vi "Config Select.vi"(0 "Config Dir":path=path "C:/Users/gtetil/Documents/Projects/TI-cDAQ/Source/Support/Configurations", 1 "Config Extension":string="*.std", 5 "Error IN":errorcluster) -> (14 "Load Config":bool, 15 "Config Name":string, 19 "Error OUT":errorcluster)   [LabVIEW 2023]
panel:
  in  "Cancel Button":bool
  in  "Load Button":bool
  in  "Config List":i32(listbox)
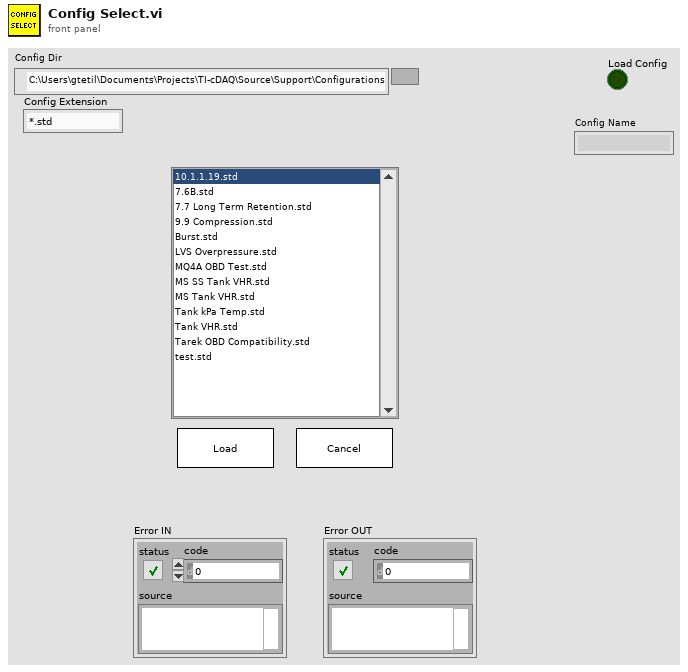
[diagram p1: front panel]
types:
  T1 = cluster{"Error IN":errorcluster, "Config Dir":path, "Config Extension":string, "Load Config":bool, "Config Name":string, "Config List":string[]}
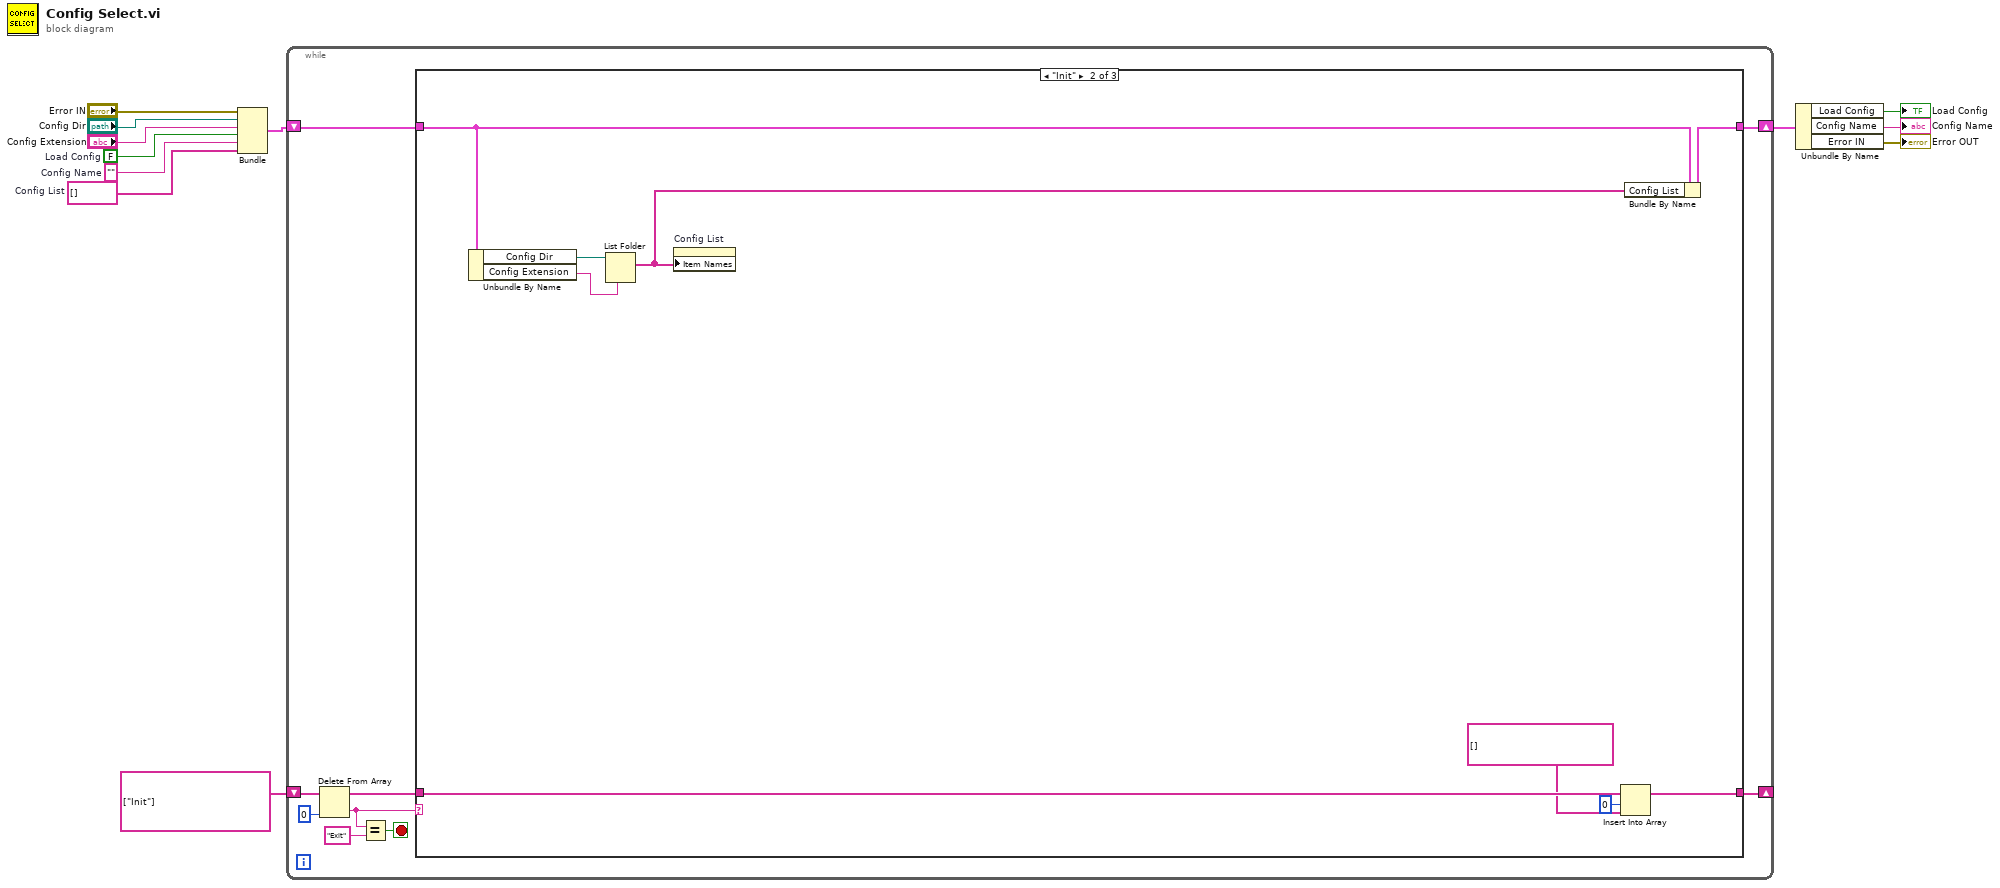
[diagram p0: block diagram]
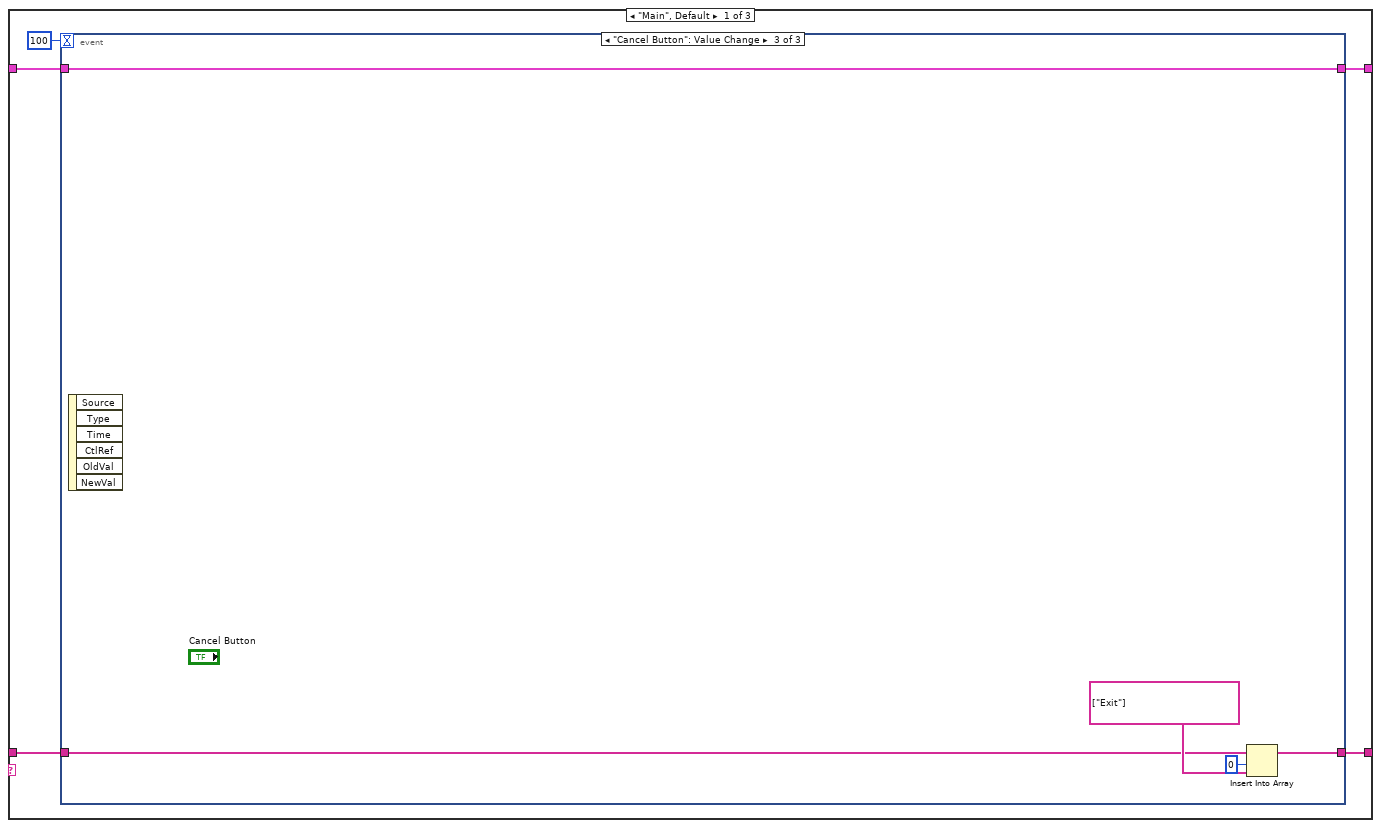
[diagram p2: hidden frame]
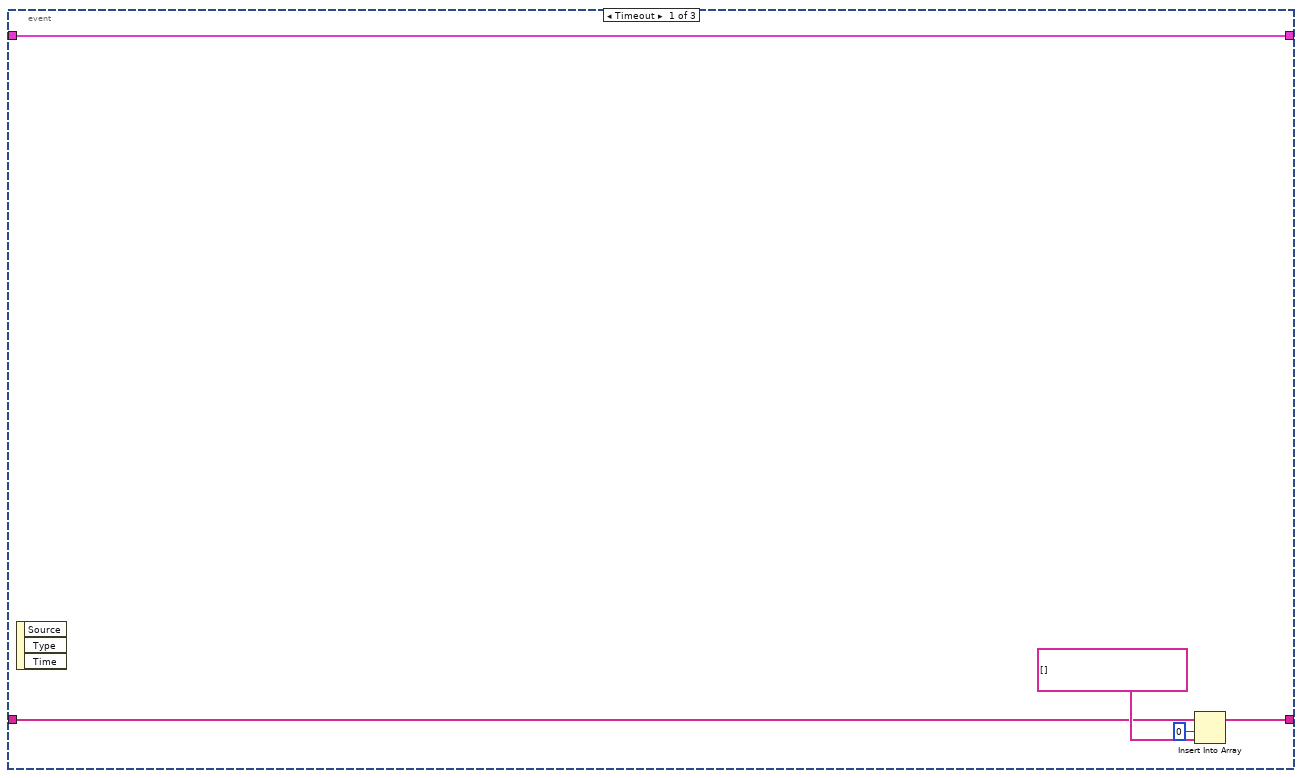
[diagram p3: hidden frame]
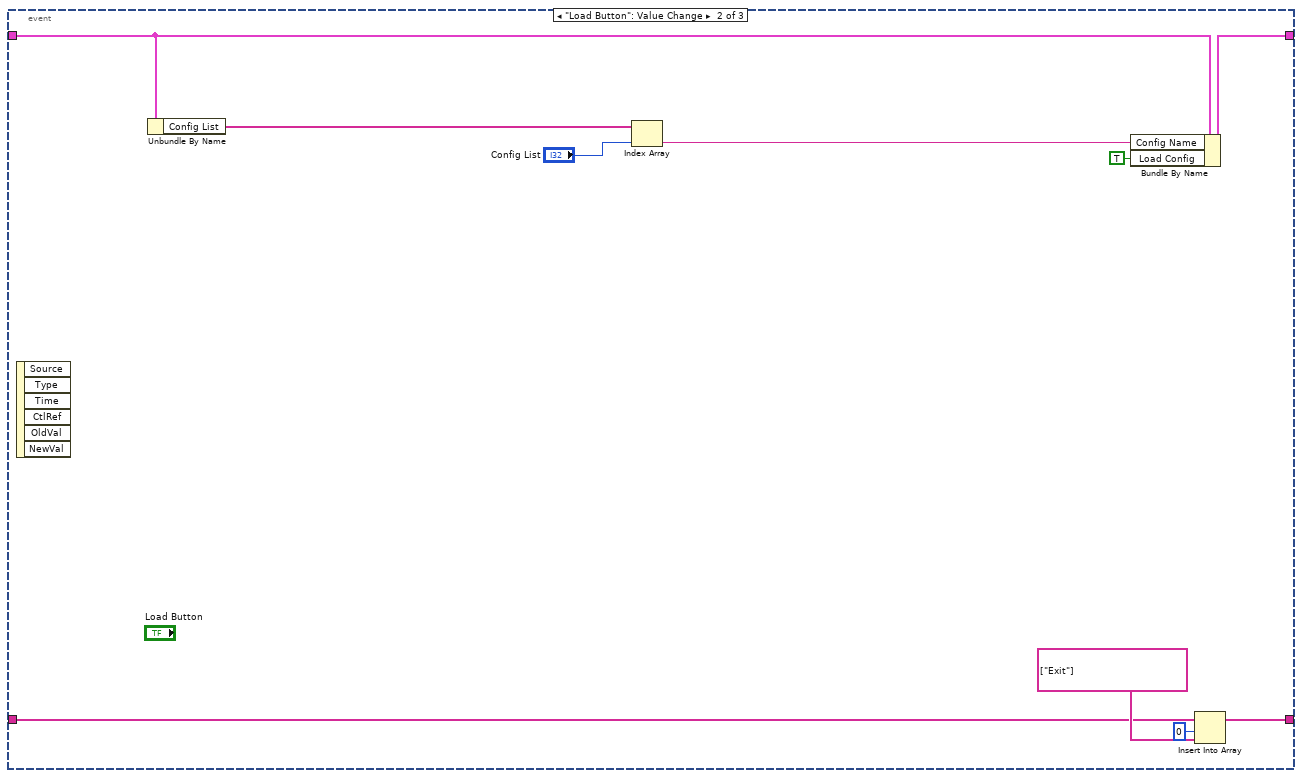
[diagram p4: hidden frame]
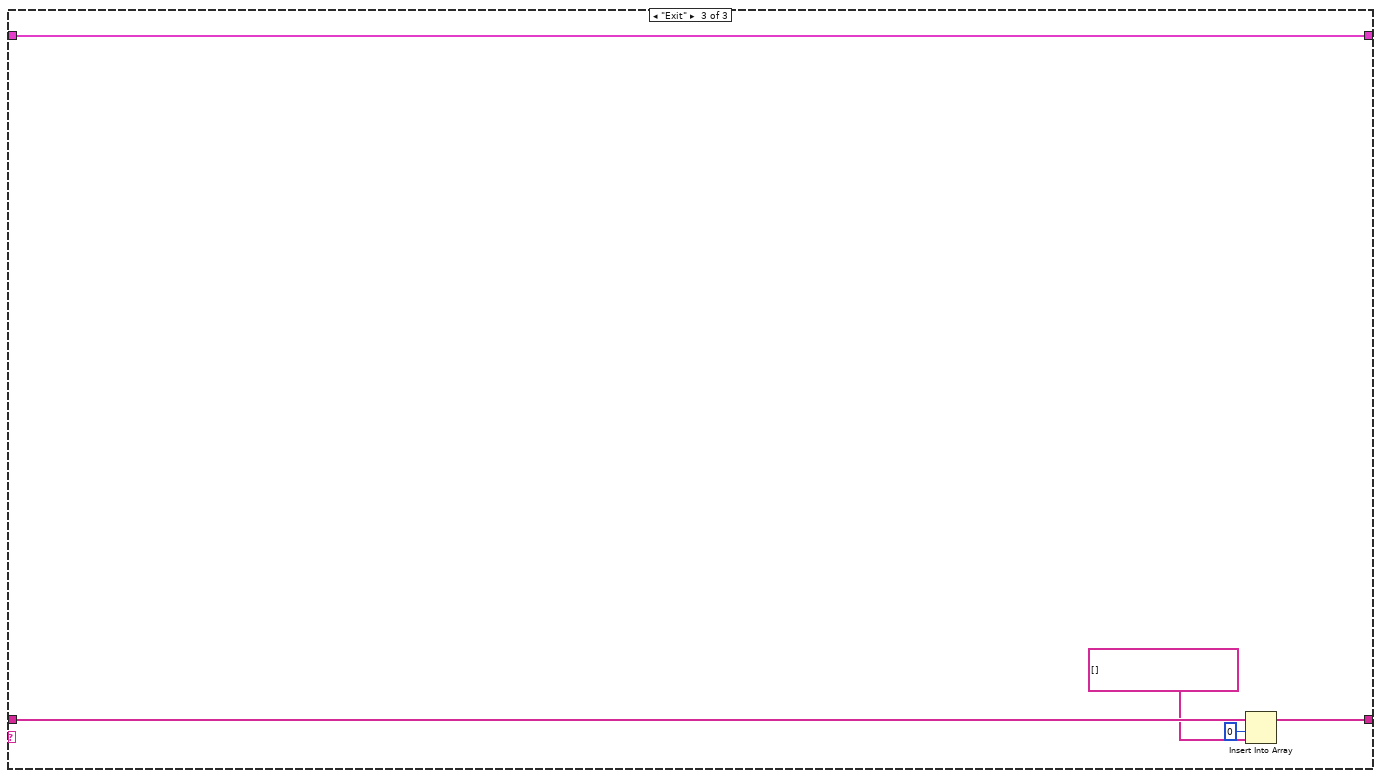
[diagram p5: hidden frame]
diagram:
  w2 = string[] []  # Config List
  w3 = ""  # Config Name
  w4 = FALSE  # Load Config
  n1 = Bundle("Error IN"="Error IN", "Config Dir"="Config Dir", "Config Extension"="Config Extension", "Load Config"=w4, "Config Name"=w3, "Config List"=w2) -> (w6:T1)  [unwired: 1 in]
  n2 = while {
    shift-right: [w16] -> _
    shift-left: string[] ["Init"] -> [w21]
    shift-right: [w13] -> w9
    shift-left: w6 -> [w14]
    stop <- w17 stop-if-true
    n3 = Delete From Array(array=w21, index=0 ("length")) -> (deleted portion=w18:string, array with subset deleted=w15:string[])  [unwired: 1 in]
    n4 = Equal?(x=w18, y="Exit") -> (x = y?=w17:bool)
    n5 = case shown="\"Init\"" w18 {
      tunnel: [w22 w55 w60] -> w16
      tunnel: w15 -> [w23 w54 w59]
      tunnel: w14 -> [w26 w48 w56]
      tunnel: [w25 w49 w56] -> w13
      frame "Main", Default {
        n6 = event shown="[2] \"Cancel Button\": Value Change" {
          selector: _ -> [_ _ _]
          dyn-events: _ -> [_ _ _]
          timeout: 100 -> [_ _ _]
          tunnel: w26 -> [w31 w36 w42]
          tunnel: [w31 w37 w42] -> w25
          tunnel: w23 -> [w28 w39 w44]
          tunnel: [w27 w38 w43] -> w22
          event Timeout {
            n7 = event-data() -> ()  [unwired: 1 in, 3 out]
            n8 = Insert Into Array(array=w28, index=0, new element=string[] []) -> (w27:string[])
          }
          event "Load Button": Value Change {
            n9 = event-data() -> ()  [unwired: 1 in, 6 out]
            n10 = Unbundle By Name(w36) -> ("Config List"=w35:string[])
            n11 = Index Array(array=w35, index="Config List") -> (element=w33:string)
            n12 = Bundle By Name(cluster=w36, "Config Name"=w33, "Load Config"=TRUE) -> (w37:T1)
            n13 = Insert Into Array(array=w39, index=0, new element=string[] ["Exit"]) -> (w38:string[])
          }
          event "Cancel Button": Value Change {
            n14 = event-data() -> ()  [unwired: 1 in, 6 out]
            n15 = Insert Into Array(array=w44, index=0, new element=string[] ["Exit"]) -> (w43:string[])
          }
        }
      }
      frame "Init" {
        n16 = Unbundle By Name(w48) -> ("Config Dir"=w51:path, "Config Extension"=w50:string)
        n17 = List Folder(path=w51, pattern=w50) -> (filenames=w47:string[])  [unwired: 2 in, 3 out]
        n18 = property on="Config List" class="LstBox (strict)"("Item Names"=w47) -> ()  [unwired: 2 in, 2 out]
        n19 = Insert Into Array(array=w54, index=0, new element=string[] []) -> (w55:string[])
        n20 = Bundle By Name(cluster=w48, "Config List"=w47) -> (w49:T1)
      }
      frame "Exit" {
        n21 = Insert Into Array(array=w59, index=0, new element=string[] []) -> (w60:string[])
      }
    }
  }
  n22 = Unbundle By Name(w9) -> ("Load Config"=→"Load Config":bool, "Config Name"=→"Config Name":string, "Error IN"=→"Error OUT":errorcluster)
